vi "Init Hardware.vi"(8 "error in (no error)":errorcluster, 11 "Cryo-Con Driver in":refnum<class "Cryo-Con Driver.lvclass">) -> (0 "error out":errorcluster, 3 "Cryo-Con Driver out":refnum<class "Cryo-Con Driver.lvclass">)   [LabVIEW 2019, in "Cryo-Con Driver.lvclass"]
uses:
  Cryo-Con Driver.lvclass
  C:/GitHub/NHMFL_Core/Libraries/Instruments/VISA Instrument/VISA Instrument.lvclass
  C:/GitHub/NHMFL_Core/Libraries/Instruments/Temperature Controller Driver/Temperature Controller Driver.lvclass
  C:/GitHub/NHMFL_Core/Libraries/Instruments/Instrument Driver/Instrument Driver.lvclass
  VISA Instrument/VISA Instrument.lvclass/VISA Instrument.ctl
  VISA Instrument/Read VISA resource.vi
  VISA Instrument/Write VISA resource.vi
  Temperature Controller Driver/Read T controller configuration.vi
  Temperature Controller Driver/Temperature Controller Driver.lvclass
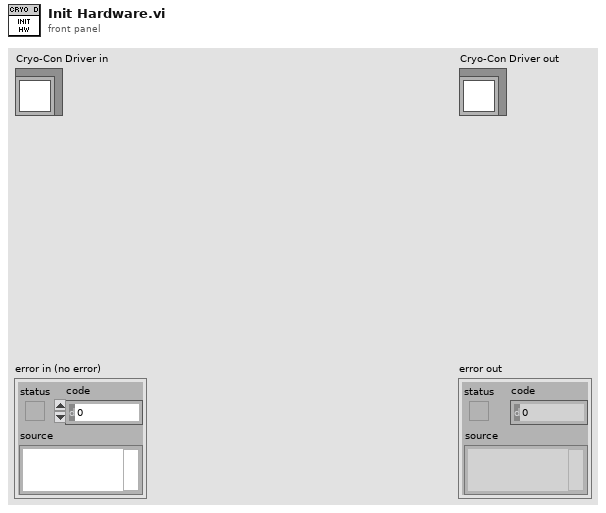
[diagram p1: front panel]
types:
  T1 = typedef "T controller configuration.ctl" = cluster{"Record Channels":string[], "Add raw signal":bool, "New set point":dbl, "Record heater":bool}
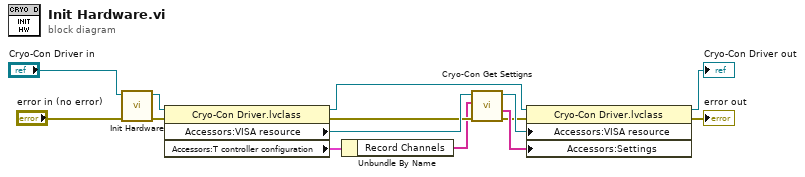
[diagram p0: block diagram]
diagram:
  n1 = call-parent "Init Hardware.vi"("error in (no error)"="error in (no error)", "Temperature Controller Driver in"="Cryo-Con Driver in") -> ("error out"=w14:errorcluster, "Temperature Controller Driver out"=w11:refnum<class "Cryo-Con Driver.lvclass">)  [unwired: 8 in]
  n2 = property class="Cryo-Con Driver.lvclass"(reference=w11, error in=w14) -> (reference out=w9:refnum<class "Cryo-Con Driver.lvclass">, error out=w4:errorcluster, "Accessors:VISA resource"=w7:refnum<visa-resource-name>, "Accessors:T controller configuration"=w2:T1)
  n3 = Unbundle By Name(w2) -> ("Record Channels"=w1:string[])
  n4 = call "Cryo-Con Get Settigns.vi"("Error In"=w4, "Inputs"=w1, "VISA resource name"=w7) -> ("Error Out"=w3:errorcluster, "Settings"=w5:string[], "VISA resource name out"=w6:refnum<visa-resource-name>)  [unwired: 6 in]
  n5 = property class="Cryo-Con Driver.lvclass"(reference=w9, error in=w3, "Accessors:VISA resource"=w6, "Accessors:Settings"=w5) -> (reference out=→"Cryo-Con Driver out":refnum<class "Cryo-Con Driver.lvclass">, error out=→"error out":errorcluster)
